vi "Mapping.vi"(0 "Ref In":refnum<vi>[](array[refnum]), 5 "SP Ref array in":refnum<vi>[](array[refnum]), 7 "Clust Refnum":refnum<vi>, 11 "error in (no error)":errorcluster) -> (4 "Ref Out":refnum<vi>[](array[refnum]), 6 "SP Ref array out":refnum<vi>[](array[refnum]), 8 "InsertedVI":refnum<vi>, 10 "SubPnl Refnum":refnum<vi>, 15 "error out":errorcluster)   [LabVIEW 2016, in "Drona basic.lvlib"]
doc: "This VI is used in Drona basic VI where to get the all elements of the cluster present"
uses:
  Drona basic.lvlib
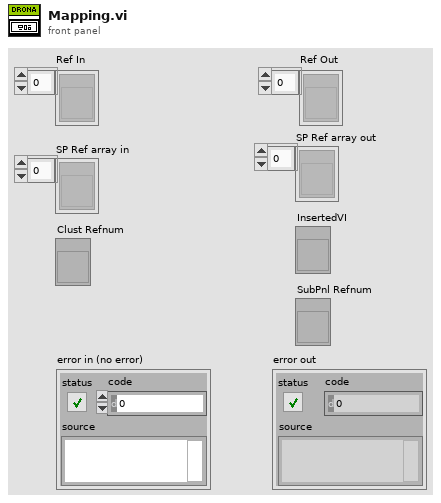
[diagram p1: front panel]
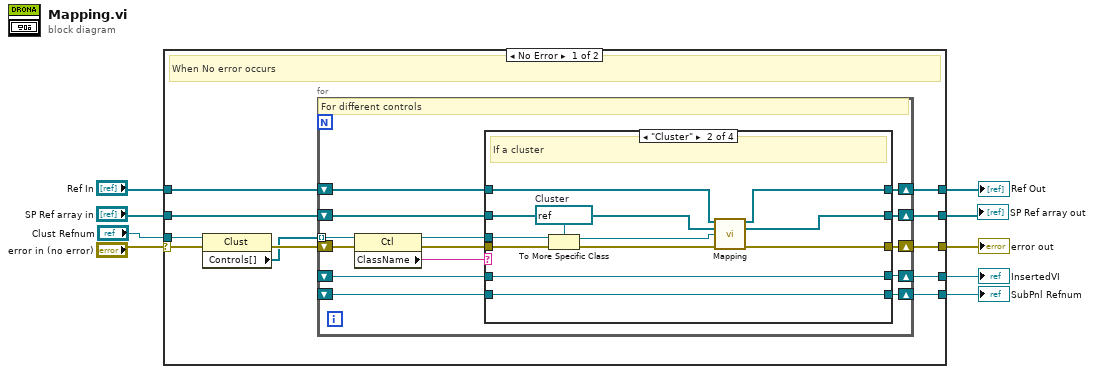
[diagram p0: block diagram]
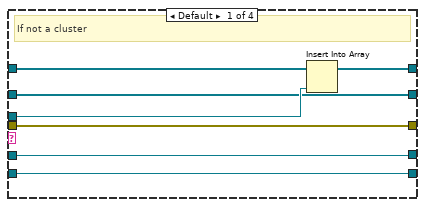
[diagram p2: hidden frame]
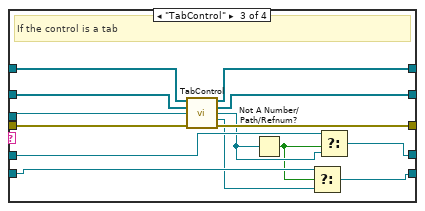
[diagram p3: hidden frame]
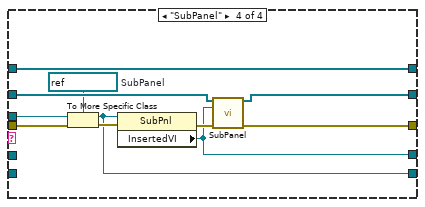
[diagram p4: hidden frame]
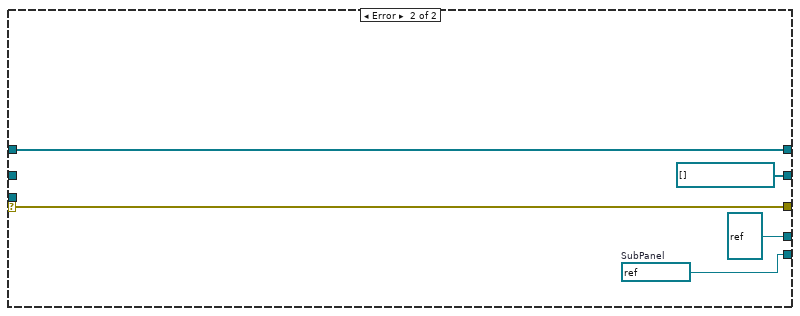
[diagram p5: hidden frame]
diagram:
  n1 = case shown="No Error" "error in (no error)" {
    selector: "error in (no error)" -> [w20 w83]
    tunnel: [w19 w83] -> w8
    tunnel: "Clust Refnum" -> [w16 _]
    tunnel: "Ref In" -> [w15 w82]
    tunnel: [w14 w82] -> w5
    tunnel: "SP Ref array in" -> [w13 _]
    tunnel: [w12 refnum<vi>[] [] ("Ref Out")] -> w3
    tunnel: [w11 refnum<vi> refnum ("InsertedVI")] -> w2
    tunnel: [w10 w79] -> w1
    frame No Error {
      # "When No error occurs"
      n2 = property class="Clust"(reference=w16, error in=w20) -> (error out=w18:errorcluster, "Controls[]"=w17:refnum<vi>[])  [unwired: 1 out]
      n3 = for {
        shift-right: [w32] -> w19
        shift-left: w18 -> [w34]
        tunnel: w17 -> [w33] mode=indexing
        shift-right: [w28] -> w14
        shift-left: w15 -> [w29]
        shift-right: [w25] -> w12
        shift-left: w13 -> [w26]
        shift-right: [w24] -> w11
        shift-left: _ -> [w22]
        shift-right: [w23] -> w10
        shift-left: _ -> [w21]
        # "For different controls"
        n4 = property class="Ctl"(reference=w33, error in=w34) -> (reference out=w30:refnum<vi>, error out=w31:errorcluster, "ClassName"=w27:string)
        n5 = case shown="\"Cluster\"" w27 {
          tunnel: [w41 w47 w66 w78] -> w32
          tunnel: w31 -> [w41 w51 w67 w73]
          tunnel: w30 -> [w39 w53 w63 w74]
          tunnel: w29 -> [w40 w49 w65 w77]
          tunnel: [w38 w48 w64 w77] -> w28
          tunnel: w26 -> [w36 w43 w62 w76]
          tunnel: [w36 w42 w61 w75] -> w25
          tunnel: [w37 w45 w54 w70] -> w24
          tunnel: [w35 w46 w55 w68] -> w23
          tunnel: w22 -> [w37 w45 w60 _]
          tunnel: w21 -> [w35 w46 w59 _]
          frame Default {
            # "If not a cluster"
            n6 = Insert Into Array(array=w40, new element=w39) -> (w38:refnum<vi>[])  [unwired: 1 in]
          }
          frame "Cluster" {
            w52 = refnum<vi> refnum  # Cluster
            # "If a cluster"
            n7 = To More Specific Class(target class=w52, reference=w53, error in=w51) -> (specific class reference=w44:refnum<vi>, error out=w50:errorcluster)
            n8 = call "Mapping.vi"("Ref In"=w49, "SP Ref array in"=w43, "Clust Refnum"=w44, "error in (no error)"=w50) -> ("Ref Out"=w48:refnum<vi>[], "SP Ref array out"=w42:refnum<vi>[], "error out"=w47:errorcluster)  [unwired: 7 in, 2 out]
          }
          frame "TabControl" {
            # "If the control is a tab"
            n9 = call "TabControl.vi"("Ref In"=w65, "SP Ref array in"=w62, "Ctl Refnum"=w63, "error in (no error)"=w67) -> ("Ref Out"=w64:refnum<vi>[], "SP Ref array out"=w61:refnum<vi>[], "InsertedVI"=w58:refnum<vi>, "SubPnl Refnum"=w56:refnum<vi>, "error out"=w66:errorcluster)  [unwired: 7 in]
            n10 = Not A Number/Path/Refnum?(number/path/refnum=w58) -> (NaN/Path/Refnum?=w57:bool)
            n11 = Select(t=w59, s=w57, f=w56) -> (s? t:f=w55:refnum<vi>)
            n12 = Select(t=w60, s=w57, f=w58) -> (s? t:f=w54:refnum<vi>)
          }
          frame "SubPanel" {
            w72 = refnum<vi> refnum  # SubPanel
            n13 = To More Specific Class(target class=w72, reference=w74, error in=w73) -> (specific class reference=w68:refnum<vi>, error out=w69:errorcluster)
            n14 = property class="SubPnl"(reference=w68, error in=w69) -> (error out=w71:errorcluster, "InsertedVI"=w70:refnum<vi>)  [unwired: 1 out]
            n15 = call "SubPanel.vi"("Ref In"=w76, "VI reference"=w70, "error in (no error)"=w71) -> ("Ref Out"=w75:refnum<vi>[], "error out"=w78:errorcluster)  [unwired: 11 in]
          }
        }
      }
    }
    frame Error {
      w79 = refnum<vi> refnum  # SubPanel
    }
  }
  "error out" <- w8
  "Ref Out" <- w5
  "InsertedVI" <- w2
  "SubPnl Refnum" <- w1
  "SP Ref array out" <- w3
